vi "Test Settings.vi"(8 "error in (no error)":errorcluster) -> (0 "error out":errorcluster)   [LabVIEW 2018, in "JSON to LVConstant Test.lvlib"]
uses:
  JSON to LVConstant Test.lvlib
  Source/SLL Scripting/DataType/_Typedefs/Settings.ctl
  Source/SLL Scripting/DataType/_Typedefs/Treat Null As.ctl
  <vilib>/numeric/LVNumericRepresentation.ctl
  <vilib>/addons/_JKI Toolkits/Caraya/classes/Assert/Assert Equal Type_Variant.vi
  <vilib>/addons/_JKI Toolkits/Caraya/classes/Test/Test.lvclass
  Source/SLL Scripting/SLL Scripting.lvlib
  <vilib>/addons/_JKI Toolkits/Caraya/classes/Assert/Assert.lvclass
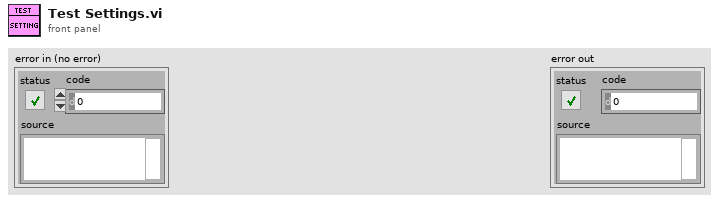
[diagram p1: front panel]
types:
  T1 = typedef "SLL Scripting.lvlib/Settings.ctl" = cluster{"Treat null as":T2, "Representation":T3}
  T2 = typedef "SLL Scripting.lvlib/Treat Null As.ctl" = enum16{"Ignore null", "Empty Object", "Empty Array", "String"}
  T3 = typedef "LVNumericRepresentation.ctl" = enum32{"Extended Precision", "Double Precision", "Single Precision", "Long", "Word", "Byte", "Unsigned Long", "Unsigned Word", "Unsigned Byte", "Complex Extended", "Complex Double", "Complex Single", "Quad", "Unsigned Quad", "Fixed-Point"}
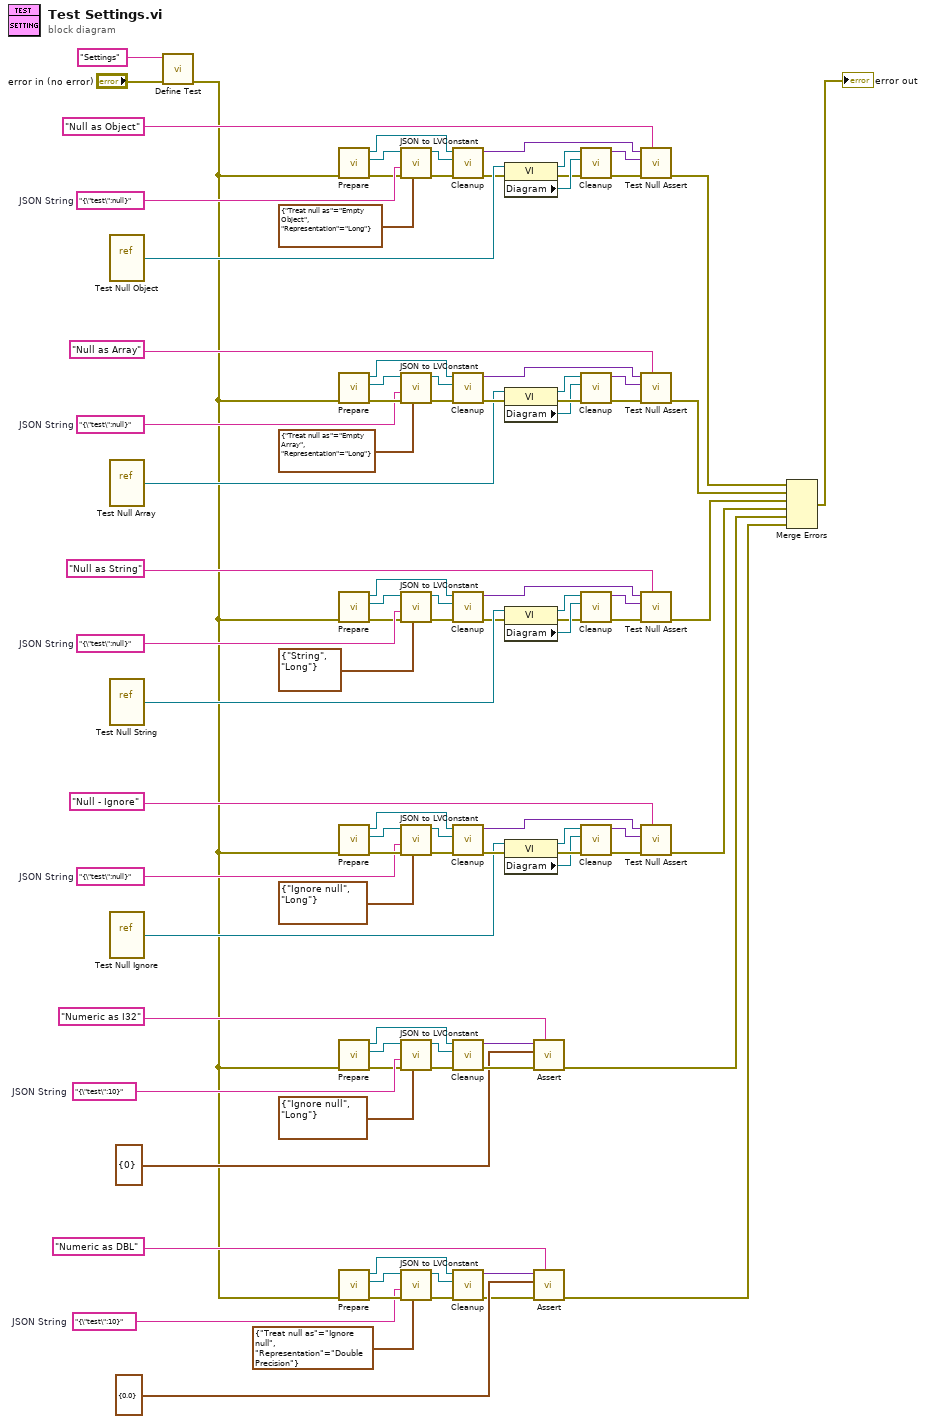
[diagram p0: block diagram]
diagram:
  w3 = "{\"test\":10}"  # JSON String
  w25 = "{\"test\":10}"  # JSON String
  w28 = "{\"test\":null}"  # JSON String
  w58 = "{\"test\":null}"  # JSON String
  w61 = "{\"test\":null}"  # JSON String
  w96 = "{\"test\":null}"  # JSON String
  n1 = vi-ref "Test Null Object.vi"() -> (w86:refnum<vi>)
  n2 = vi-ref "Test Null Array.vi"() -> (w60:refnum<vi>)
  n3 = vi-ref "Test Null String.vi"() -> (w59:refnum<vi>)
  n4 = vi-ref "Test Null Ignore.vi"() -> (w27:refnum<vi>)
  n5 = call <vilib>:"Define Test.vi"("error in (no error)"="error in (no error)", "Label (VI Title)"="Settings") -> ("error out"=w1:errorcluster)  [unwired: 9 in]
  n6 = call "Prepare.vi"("error in (no error)"=w1) -> ("error out"=w91:errorcluster, "Owner"=w90:refnum<vi>, "vi refnum"=w89:refnum<vi>)  [unwired: 8 in]
  n7 = call "Prepare.vi"("error in (no error)"=w1) -> ("error out"=w65:errorcluster, "Owner"=w66:refnum<vi>, "vi refnum"=w67:refnum<vi>)  [unwired: 8 in]
  n8 = call "Prepare.vi"("error in (no error)"=w1) -> ("error out"=w55:errorcluster, "Owner"=w54:refnum<vi>, "vi refnum"=w53:refnum<vi>)  [unwired: 8 in]
  n9 = call "Prepare.vi"("error in (no error)"=w1) -> ("error out"=w31:errorcluster, "Owner"=w32:refnum<vi>, "vi refnum"=w33:refnum<vi>)  [unwired: 8 in]
  n10 = call "Prepare.vi"("error in (no error)"=w1) -> ("error out"=w22:errorcluster, "Owner"=w21:refnum<vi>, "vi refnum"=w20:refnum<vi>)  [unwired: 8 in]
  n11 = call "Prepare.vi"("error in (no error)"=w1) -> ("error out"=w6:errorcluster, "Owner"=w7:refnum<vi>, "vi refnum"=w8:refnum<vi>)  [unwired: 8 in]
  n12 = call "JSON to LVConstant.vi"("Settings"=T1 {"Treat null as"=enum."Empty Object", "Representation"=enum."Long"}, "error in (no error)"=w91, "<JSON>"=w96, "owner refnum in"=w90) -> ("error out"=w92:errorcluster, "owner refnum out"=w88:refnum<vi>)  [unwired: 6 in]
  n13 = call "JSON to LVConstant.vi"("Settings"=T1 {"Treat null as"=enum."Empty Array", "Representation"=enum."Long"}, "error in (no error)"=w65, "<JSON>"=w61, "owner refnum in"=w66) -> ("error out"=w64:errorcluster, "owner refnum out"=w68:refnum<vi>)  [unwired: 6 in]
  n14 = call "JSON to LVConstant.vi"("Settings"=T1 {"Treat null as"=enum."String", "Representation"=enum."Long"}, "error in (no error)"=w55, "<JSON>"=w58, "owner refnum in"=w54) -> ("error out"=w56:errorcluster, "owner refnum out"=w52:refnum<vi>)  [unwired: 6 in]
  n15 = call "JSON to LVConstant.vi"("Settings"=T1 {"Treat null as"=enum."Ignore null", "Representation"=enum."Long"}, "error in (no error)"=w31, "<JSON>"=w28, "owner refnum in"=w32) -> ("error out"=w30:errorcluster, "owner refnum out"=w34:refnum<vi>)  [unwired: 6 in]
  n16 = call "JSON to LVConstant.vi"("Settings"=T1 {"Treat null as"=enum."Ignore null", "Representation"=enum."Long"}, "error in (no error)"=w22, "<JSON>"=w25, "owner refnum in"=w21) -> ("error out"=w23:errorcluster, "owner refnum out"=w19:refnum<vi>)  [unwired: 6 in]
  n17 = call "JSON to LVConstant.vi"("Settings"=T1 {"Treat null as"=enum."Ignore null", "Representation"=enum."Double Precision"}, "error in (no error)"=w6, "<JSON>"=w3, "owner refnum in"=w7) -> ("error out"=w5:errorcluster, "owner refnum out"=w9:refnum<vi>)  [unwired: 6 in]
  n18 = call "Cleanup.vi"("error in (no error)"=w92, "Owner"=w88, "vi refnum"=w89) -> ("error out"=w80:errorcluster, "Type out"=w77:variant)  [unwired: 7 in]
  n19 = call "Cleanup.vi"("error in (no error)"=w64, "Owner"=w68, "vi refnum"=w67) -> ("error out"=w73:errorcluster, "Type out"=w76:variant)  [unwired: 7 in]
  n20 = call "Cleanup.vi"("error in (no error)"=w56, "Owner"=w52, "vi refnum"=w53) -> ("error out"=w47:errorcluster, "Type out"=w44:variant)  [unwired: 7 in]
  n21 = call "Cleanup.vi"("error in (no error)"=w30, "Owner"=w34, "vi refnum"=w33) -> ("error out"=w39:errorcluster, "Type out"=w42:variant)  [unwired: 7 in]
  n22 = call "Cleanup.vi"("error in (no error)"=w23, "Owner"=w19, "vi refnum"=w20) -> ("error out"=w18:errorcluster, "Type out"=w16:variant)  [unwired: 7 in]
  n23 = call "Cleanup.vi"("error in (no error)"=w5, "Owner"=w9, "vi refnum"=w8) -> ("error out"=w10:errorcluster, "Type out"=w12:variant)  [unwired: 7 in]
  n24 = property class="VI"(reference=w86, error in=w80) -> (reference out=w85:refnum<vi>, error out=w83:errorcluster, "Diagram"=w84:refnum<vi>)
  n25 = property class="VI"(reference=w60, error in=w73) -> (reference out=w69:refnum<vi>, error out=w71:errorcluster, "Diagram"=w70:refnum<vi>)
  n26 = property class="VI"(reference=w59, error in=w47) -> (reference out=w51:refnum<vi>, error out=w49:errorcluster, "Diagram"=w50:refnum<vi>)
  n27 = property class="VI"(reference=w27, error in=w39) -> (reference out=w35:refnum<vi>, error out=w37:errorcluster, "Diagram"=w36:refnum<vi>)
  n28 = call-poly <vilib>:"Assert.vi"("Label"="Numeric as I32" ("Label (VI Title)"), "error in (no error)"=w18, "Y"=cluster{"test":i32} {"test"=0}, "X"=w16) -> ("error out"=w15:errorcluster)  [unwired: 7 in]
  n29 = call-poly <vilib>:"Assert.vi"("Label"="Numeric as DBL" ("Label (VI Title)"), "error in (no error)"=w10, "Y"=cluster{"test":dbl} {"test"=0.0}, "X"=w12) -> ("error out"=w2:errorcluster)  [unwired: 7 in]
  n30 = call "Cleanup.vi"("error in (no error)"=w83, "Owner"=w84, "vi refnum"=w85) -> ("error out"=w79:errorcluster, "Type out"=w78:variant)  [unwired: 7 in]
  n31 = call "Cleanup.vi"("error in (no error)"=w71, "Owner"=w70, "vi refnum"=w69) -> ("error out"=w74:errorcluster, "Type out"=w75:variant)  [unwired: 7 in]
  n32 = call "Cleanup.vi"("error in (no error)"=w49, "Owner"=w50, "vi refnum"=w51) -> ("error out"=w46:errorcluster, "Type out"=w45:variant)  [unwired: 7 in]
  n33 = call "Cleanup.vi"("error in (no error)"=w37, "Owner"=w36, "vi refnum"=w35) -> ("error out"=w40:errorcluster, "Type out"=w41:variant)  [unwired: 7 in]
  n34 = call "Test Null Assert.vi"("Label (VI Title)"="Null as Object", "error in (no error)"=w79, 10:"Type in"=w78, 11:"Type in"=w77) -> ("error out"=w87:errorcluster)  [unwired: 7 in]
  n35 = call "Test Null Assert.vi"("Label (VI Title)"="Null as Array", "error in (no error)"=w74, 10:"Type in"=w75, 11:"Type in"=w76) -> ("error out"=w63:errorcluster)  [unwired: 7 in]
  n36 = call "Test Null Assert.vi"("Label (VI Title)"="Null as String", "error in (no error)"=w46, 10:"Type in"=w45, 11:"Type in"=w44) -> ("error out"=w43:errorcluster)  [unwired: 7 in]
  n37 = call "Test Null Assert.vi"("Label (VI Title)"="Null - Ignore", "error in (no error)"=w40, 10:"Type in"=w41, 11:"Type in"=w42) -> ("error out"=w26:errorcluster)  [unwired: 7 in]
  n38 = Merge Errors(w87, w63, w43, w26, w15, w2) -> (→"error out":errorcluster)
